vi "Concatenate Waveform.vi"(5 "Base Waveform":waveform(dbl), 9 "Waveform":waveform(dbl)) -> (8 "Concatenated Waveform":waveform(dbl))   [LabVIEW 2013]
panel:
  out "Concatenated Waveform":waveform(dbl)(graph)
  out "Waveform":waveform(dbl)(graph)
  out "Base Waveform":waveform(dbl)(graph)
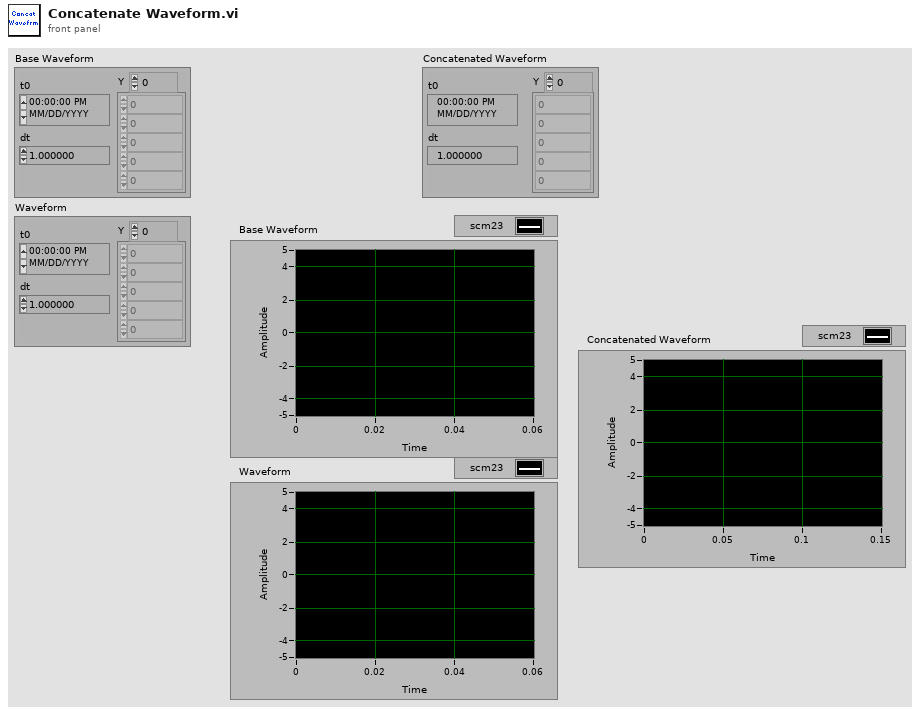
[diagram p1: front panel]
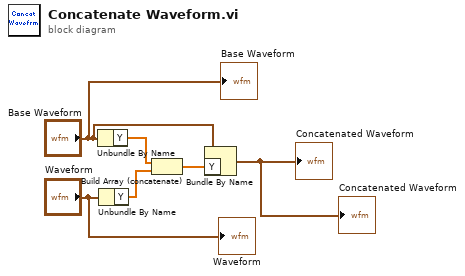
[diagram p0: block diagram]
diagram:
  n1 = Unbundle By Name("Base Waveform") -> ("Y"=w6:dbl[])
  n2 = Unbundle By Name("Waveform") -> ("Y"=w5:dbl[])
  n3 = Build Array (concatenate)(w6, w5) -> (w4:dbl[])
  n4 = Bundle By Name(cluster="Base Waveform", "Y"=w4) -> (→"Concatenated Waveform" →"Concatenated Waveform":waveform(dbl))
  "Base Waveform" <- "Base Waveform"
  "Waveform" <- "Waveform"
